vi "Defer.vi"(8 "error in (no error)":errorcluster, 11 "Deferer in":refnum<class "Deferer.lvclass">) -> (0 "error out":errorcluster, 3 "Deferer out":refnum<class "Deferer.lvclass">)   [LabVIEW 2017, in "MGI-Panel Manager.lvlib" / "Deferer.lvclass"]
doc: "Defers panel updates for the owned VI.\n\n----\nPlease see the following web address for additional documentation and tutorial information:\nhttp://www.mooregoodideas.com/mgi-panel-manager/\n\nAuthor: Derek Trepanier\n\nCopyright (c) 2018, Moore Good Ideas, Inc.\n\nAll rights reserved.\n\nRedistribution and use in source and binary forms, with or without modification, are permitted provided that the following conditions are met:\n\n * Redistributions of source code must retain the above copyright notice, this list of conditions and the following disclaimer.\n * Redistributions in binary form must reproduce the above copyright notice, this list of conditions and the following disclaimer in the documentation and/or other materials provided with the distribution.\n * Neither the name of Moore Good Ideas, Inc. nor the names of its contributors may be used to endorse or promote products derived from this software without specific prior written permission.\n\nTHIS SOFTWARE IS PROVIDED BY THE COPYRIGHT HOLDERS AND CONTRIBUTORS \"AS IS\" AND ANY EXPRESS OR IMPLIED WARRANTIES, INCLUDING, BUT NOT LIMITED TO, THE IMPLIED WARRANTIES OF MERCHANTABILITY AND FITNESS FOR A PARTICULAR PURPOSE ARE DISCLAIMED. IN NO EVENT SHALL THE COPYRIGHT OWNER OR CONTRIBUTORS BE LIABLE FOR ANY DIRECT, INDIRECT, INCIDENTAL, SPECIAL, EXEMPLARY, OR CONSEQUENTIAL DAMAGES (INCLUDING, BUT NOT LIMITED TO, PROCUREMENT OF SUBSTITUTE GOODS OR SERVICES; LOSS OF USE, DATA, OR PROFITS; OR BUSINESS INTERRUPTION) HOWEVER CAUSED AND ON ANY THEORY OF LIABILITY, WHETHER IN CONTRACT, STRICT LIABILITY, OR TORT (INCLUDING NEGLIGENCE OR OTHERWISE) ARISING IN ANY WAY OUT OF THE USE OF THIS SOFTWARE, EVEN IF ADVISED OF THE POSSIBILITY OF SUCH DAMAGE."
uses:
  Deferer.lvclass
  Deferer.lvclass/Deferer.ctl
  Panel Control Counter/Panel Control Counter.lvclass
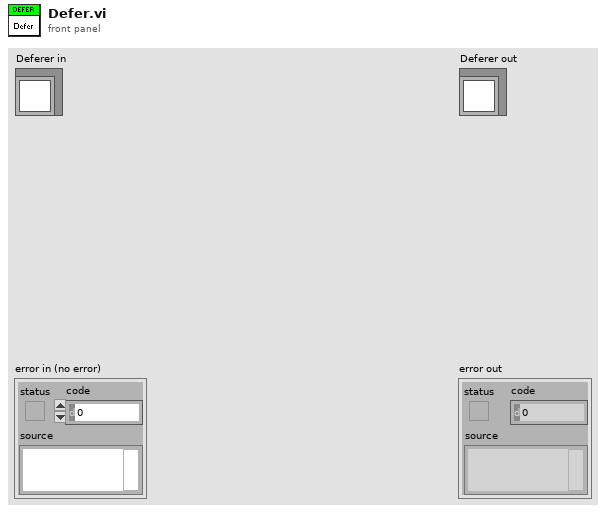
[diagram p1: front panel]
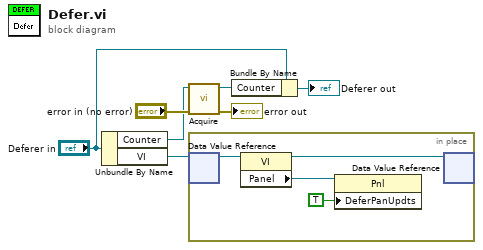
[diagram p0: block diagram]
diagram:
  n1 = Unbundle By Name("Deferer in") -> ("Counter"=w3:refnum<class "Panel Control Counter.lvclass">, "VI"=w4:refnum<data-value>)
  n2 = call "Acquire.vi"("error in (no error)"="error in (no error)", "Panel Control Counter in"=w3) -> ("error out"=→"error out":errorcluster, "Panel Control Counter out"=w1:refnum<class "Panel Control Counter.lvclass">)  [unwired: 8 in]
  n3 = in-place {
    n4 = in-place-dvr #1(w4) -> (w11:refnum<vi>)  [unwired: 1 out]
    n5 = property class="VI"(reference=w11) -> (reference out=w10:refnum<vi>, "Panel"=w9:refnum<vi>)  [unwired: 1 in, 1 out]
    n6 = property class="Pnl"(reference=w9, "DeferPanUpdts"=TRUE ("Defer Panel Updates")) -> ()  [unwired: 1 in, 2 out]
    n7 = in-place-dvr #1(w10) -> ()  [unwired: 2 out]
  }
  n8 = Bundle By Name(cluster="Deferer in", "Counter"=w1) -> (→"Deferer out":refnum<class "Deferer.lvclass">)
